vi "FTW-SQLite-CreateEphemeralDatabase.vi"(0 "Database Type":T1=enum."Memory", 11 "error in":errorcluster) -> (4 "SQLite Connector":refnum<class "FTW-SQLite-Connector.lvclass">, 15 "error out":errorcluster)   [LabVIEW 2013, in "FTW-SQLite-Connector.lvclass"]
uses:
  FTW-SQLite-Connector.lvclass
  FTW-SQLite-DatabaseType.ctl
  FTW-SQLite-AccessMode.ctl
panel:
  # "Inputs"
  # "Outputs"
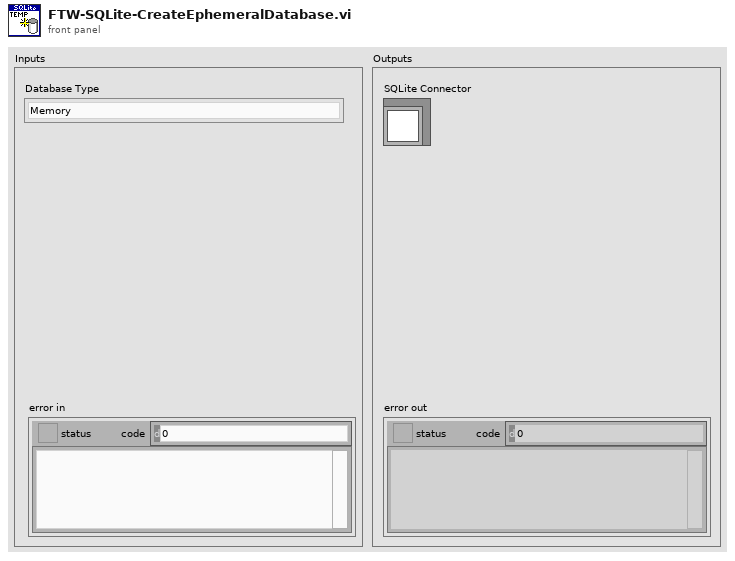
[diagram p1: front panel]
types:
  T1 = typedef "FTW-SQLite-Connector.lvclass/FTW-SQLite-DatabaseType.ctl" = enum16{"Disk", "Memory"}
  T2 = typedef "FTW-SQLite-Connector.lvclass/FTW-SQLite-AccessMode.ctl" = enum16{"Read", "Read/Write", "Read/Write/Create"}
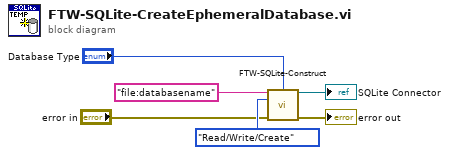
[diagram p0: block diagram]
diagram:
  n1 = call "FTW-SQLite-Construct.vi"("Database URI"="file:databasename", "Database Type"="Database Type", "Access Mode"=FTW-SQLite-AccessMode."Read/Write/Create", "error in"="error in") -> ("SQLite Connector"=→"SQLite Connector":refnum<class "FTW-SQLite-Connector.lvclass">, "error out"=→"error out":errorcluster)  [unwired: 9 in, 1 out]
